vi "CTRE_Phoenix_CANcoder_SetStatusFrameRate.vi"(6 "timeoutMs":u32, 8 "error in (no error)":errorcluster, 9 "Period (ms)":u8, 10 "CANcoder Status Frame":T1=267264 items=["SensorData"=267264, "VbatAndFaults"=267328], 11 "CTRE_CANcoder_DeviceRef":T2) -> (0 "error out":errorcluster, 3 "CTRE_CANcoder_DeviceRef":T2)   [LabVIEW 2019]
doc: "Period (ms) sets the rate at which StatusFrame is sent."
uses:
  <vilib>/Rock Robotics/WPI/ThirdParty/Phoenix-LabVIEW/CANCoder/Controls/CTRE_Phoenix_CANcoder_DeviceRef.ctl
  <vilib>/Rock Robotics/WPI/ThirdParty/Phoenix-LabVIEW/CANCoder/Controls/CTRE_Phoenix_CANcoder_StatusFrame.ctl
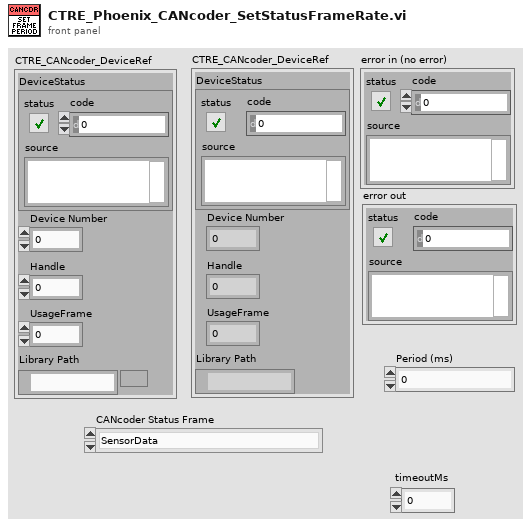
[diagram p1: front panel]
types:
  T1 = typedef "CTRE_Phoenix_CANcoder_StatusFrame.ctl" = u32
  T2 = typedef "CTRE_Phoenix_CANcoder_DeviceRef.ctl" = cluster{"DeviceStatus":errorcluster, "Device Number":u8, "Handle":u64, "UsageFrame":u32, "Library Path":path}
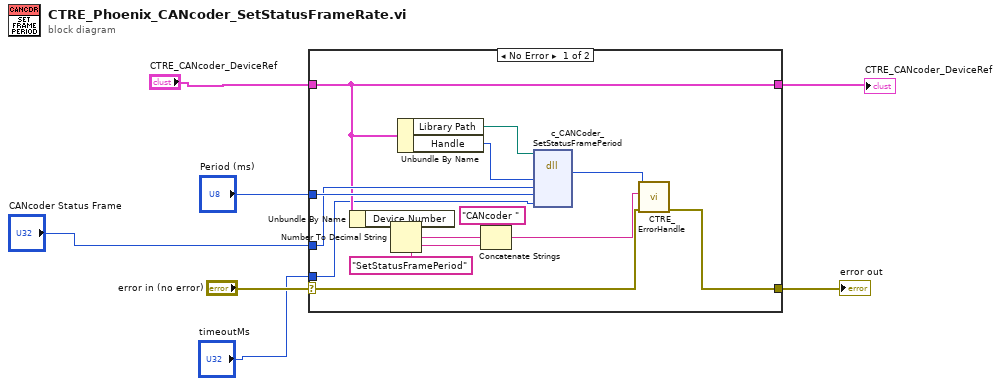
[diagram p0: block diagram]
diagram:
  n1 = case shown="No Error" "error in (no error)" {
    selector: "error in (no error)" -> [w10 w22]
    tunnel: [w9 w22] -> w6
    tunnel: [w12 w23] -> w2
    tunnel: "CTRE_CANcoder_DeviceRef" -> [w12 w23]
    tunnel: "Period (ms)" -> [w19 _]
    tunnel: "CANcoder Status Frame" -> [w18 _]
    tunnel: "timeoutMs" -> [w8 _]
    frame No Error {
      n2 = Unbundle By Name(w12) -> ("Device Number"=w16:u8)
      n3 = Number To Decimal String(number=w16) -> (decimal integer string=w15:string)  [unwired: 1 in]
      n4 = Unbundle By Name(w12) -> ("Library Path"=w21:path, "Handle"=w20:u64)
      n5 = Concatenate Strings("CANcoder " ("string"), w15, "SetStatusFramePeriod" ("string")) -> (w11:string)
      n6 = dll-call lib="?" fn="c_CANCoder_SetStatusFramePeriod"(path in=w21, "handle"=w20, "statusFrame"=w18, "periodMs"=w19, "timeoutms"=w8) -> ("return type"=w17:i32)  [unwired: 6 in, 2 out]
      n7 = call <vilib>:"CTRE_ErrorHandle.vi"("error in"=w10, "origin"=w11, "code"=w17) -> ("error out"=w9:errorcluster)  [unwired: 8 in]
    }
    frame Error {
    }
  }
  "error out" <- w6
  "CTRE_CANcoder_DeviceRef" <- w2
